vi "CheckHit.vi"(0 "object in":refnum<class "Battleship.lvclass">, 2 "Shot\nCoordinates":T1, 5 "error in (no error)":errorcluster) -> (14 "object out":refnum<class "Battleship.lvclass">, 16 "Hit?":bool, 19 "error out":errorcluster)   [LabVIEW 2015, in "Battleship.lvclass"]
doc: "Returns true if the ship was hit by the shot defined by the ShotCoordinates input."
uses:
  Battleship.lvclass
  TypDefs/Coordinates.ctl
  Battleship.lvclass/Battleship.ctl
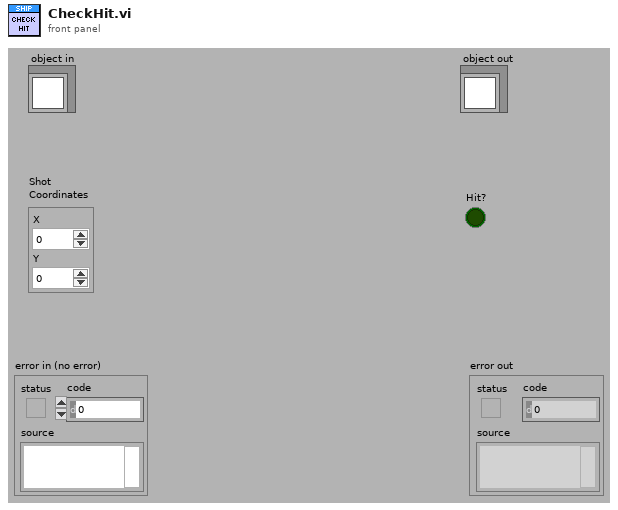
[diagram p1: front panel]
types:
  T1 = typedef "Coordinates.ctl" = cluster{"X":i32, "Y":i32}
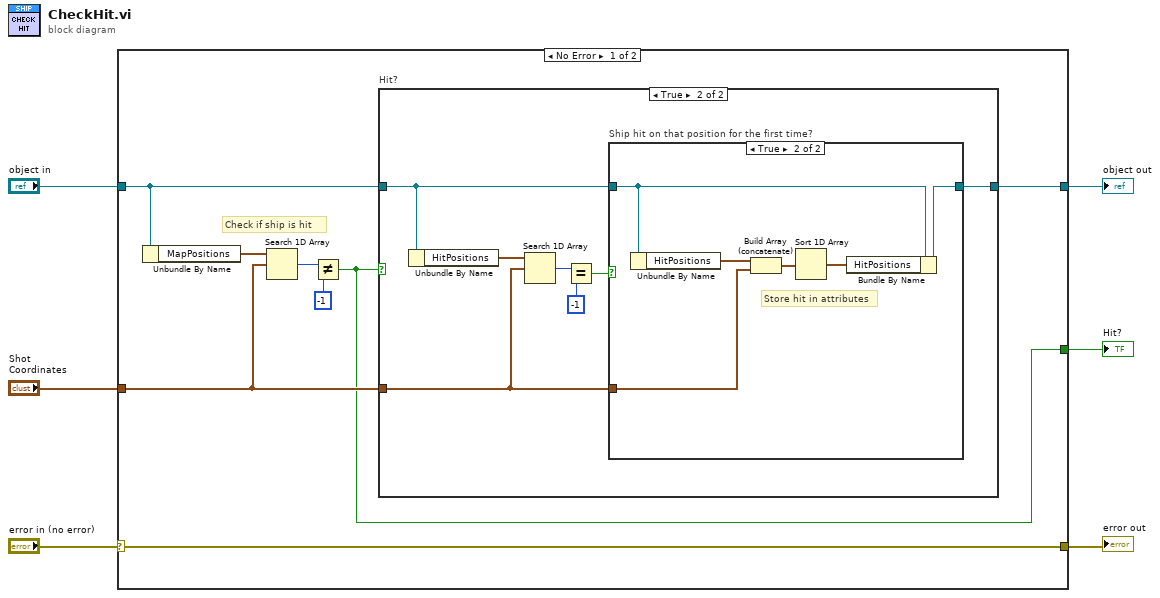
[diagram p0: block diagram]
diagram:
  n1 = case shown="No Error" "error in (no error)" {
    selector: "error in (no error)" -> [w8 w31]
    tunnel: [w8 w31] -> w5
    tunnel: [w7 w30] -> w3
    tunnel: "object in" -> [w11 w30]
    tunnel: "Shot\nCoordinates" -> [w10 _]
    tunnel: [w9 _] -> w1
    frame No Error {
      # "Check if ship is hit"
      n2 = Unbundle By Name(w11) -> ("MapPositions"=w14:T1[])
      n3 = Search 1D Array(1D array=w14, element=w10) -> (index of element=w13:i32)  [unwired: 1 in]
      n4 = Not Equal?(x=w13, y=-1) -> (x != y?=w9:bool)
      n5 = case "Hit?" shown="True" w9 {
        tunnel: w11 -> [w15 w18]
        tunnel: [w15 w19] -> w7
        tunnel: w10 -> [_ w16]
        frame False {
        }
        frame True {
          n6 = Unbundle By Name(w18) -> ("HitPositions"=w20:T1[])
          n7 = Search 1D Array(1D array=w20, element=w16) -> (index of element=w21:i32)  [unwired: 1 in]
          n8 = Equal?(x=w21, y=-1) -> (x = y?=w17:bool)
          n9 = case "Ship hit on that position for the first time?" shown="True" w17 {
            tunnel: [w23 w26] -> w19
            tunnel: w18 -> [w23 w29]
            tunnel: w16 -> [_ w27]
            frame False {
              # "Ship was already hit on that position"
            }
            frame True {
              # "Store hit in attributes"
              n10 = Unbundle By Name(w29) -> ("HitPositions"=w28:T1[])
              n11 = Build Array (concatenate)(w28, w27) -> (w25:T1[])
              n12 = Sort 1D Array(array=w25) -> (sorted array=w24:T1[])
              n13 = Bundle By Name(cluster=w29, "HitPositions"=w24) -> (w26:refnum<class "Battleship.lvclass">)
            }
          }
        }
      }
    }
    frame Error {
    }
  }
  "error out" <- w5
  "object out" <- w3
  "Hit?" <- w1
